vi "Is IO Read State Ready.vi"() -> (3 "function return":i32)   [LabVIEW 2021, in "vmmso.lvlib"]
doc: "DLL_API int WINAPI IsIOReadStateReady();"
uses:
  vmmso.lvlib
  vmmso.dll
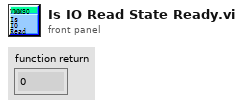
[diagram p1: front panel]
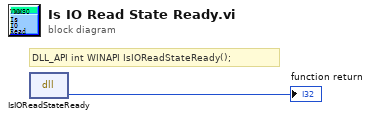
[diagram p0: block diagram]
diagram:
  # "DLL_API int WINAPI IsIOReadStateReady();"
  n1 = dll-call lib="D:/labviewdemo/LabviewDemo 21/vmmso/vmmso.*" fn="IsIOReadStateReady"() -> (→"function return":i32)  [unwired: 3 in, 2 out]
